vi "ReadMatlabMessagesFromTempID.vi"(10 "Numeric":dbl, 11 "ExperimentID":string) -> (3 "Read messages":T1[](array[typedef]))   [LabVIEW 2017]
uses:
  Types/MatlabEventStruct.ctl
  Types/MatlabDataBundle.ctl
  Types/MatlabDataType.ctl
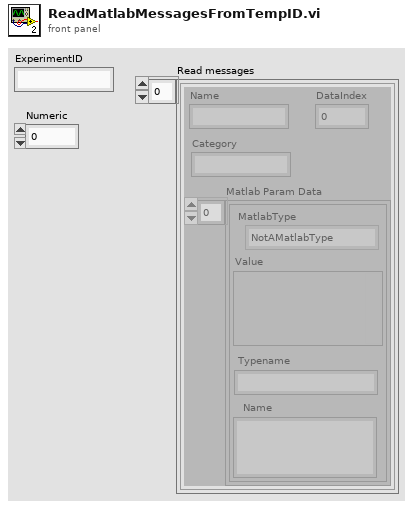
[diagram p1: front panel]
types:
  T1 = typedef "MatlabEventStruct.ctl" = cluster{"Name":string, "DataIndex":dbl, "Category":string, "Matlab Param Data":T2[]}
  T2 = typedef "MatlabDataBundle.ctl" = cluster{"MatlabType":T3, "Value":variant, "Name":string, "Typename":string}
  T3 = typedef "MatlabDataType.ctl" = enum16{"NotAMatlabType", "Real", "Complex", "String", "Boolean"}
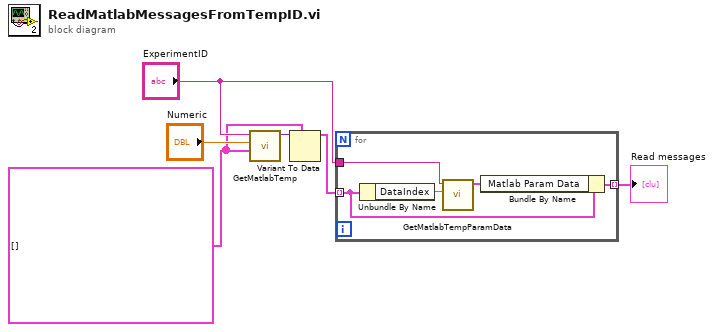
[diagram p0: block diagram]
diagram:
  w2 = T1[] []
  n1 = call "GetMatlabTemp.vi"("Value To Update (or type)"=w2, "index in"="Numeric", "ExpID"="ExperimentID") -> ("Value"=w6:variant)  [unwired: 6 in, 2 out]
  n2 = Variant To Data(type=w2, Variant=w6) -> (data=w3:T1[])  [unwired: 1 in, 1 out]
  n3 = for {
    tunnel: w3 -> [w8] mode=indexing
    tunnel: [w11] -> w1 mode=indexing
    tunnel: "ExperimentID" -> [w10]
    n4 = Unbundle By Name(w8) -> ("DataIndex"=w7:dbl)
    n5 = call "GetMatlabTempParamData.vi"("index"=w7, "ExpID"=w10) -> ("Matlab param data"=w9:T2[])  [unwired: 9 in]
    n6 = Bundle By Name(cluster=w8, "Matlab Param Data"=w9) -> (w11:T1)
  }
  "Read messages" <- w1
